vi "Min phase set (SubVI).vi"(3 "pos_z":dbl, 4 "error in":errorcluster, 5 "step search":i32=50, 6 "set_pos_min":dbl, 7 "VISA Refnum in":refnum<visa-resource-name>) -> (0 "error out":errorcluster, 1 "Min phase":dbl)   [LabVIEW 2018]
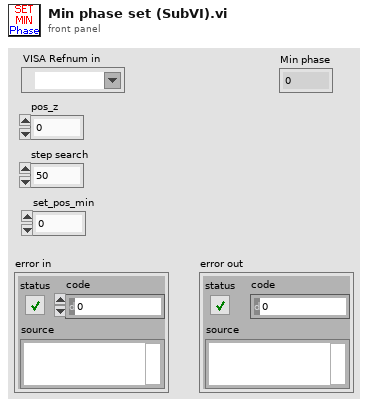
[diagram p1: front panel]
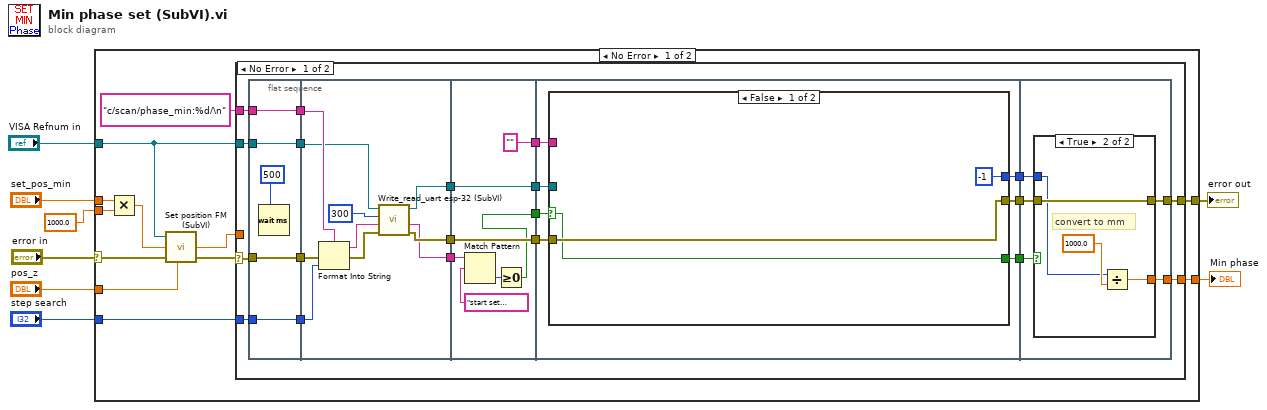
[diagram p0: block diagram]
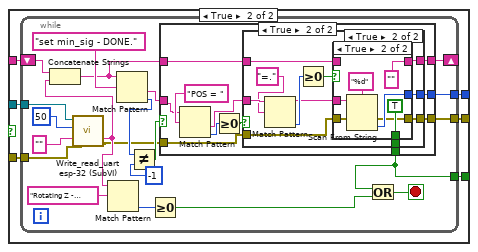
[diagram p2: hidden frame]
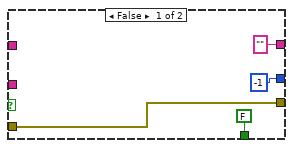
[diagram p3: hidden frame]
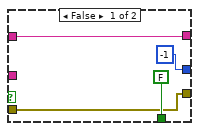
[diagram p4: hidden frame]
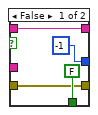
[diagram p5: hidden frame]
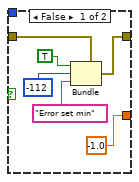
[diagram p6: hidden frame]
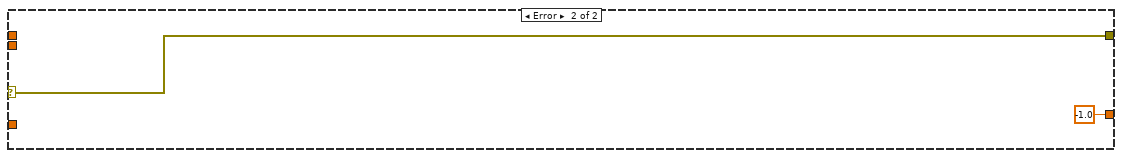
[diagram p8: hidden frame]
diagram:
  n1 = case shown="No Error" "error in" {
    selector: "error in" -> [w16 w159]
    tunnel: "VISA Refnum in" -> [w17 _]
    tunnel: [w20 w159] -> w8
    tunnel: [w19 -1.0] -> w5
    tunnel: "step search" -> [w18 _]
    tunnel: "pos_z" -> [w13 _]
    tunnel: "set_pos_min" -> [w12 _]
    tunnel: 1000.0 ("y") -> [w9 _]
    frame No Error {
      n2 = Multiply(x=w12, y=w9) -> (x*y=w11:dbl)
      n3 = call "Set position FM (SubVI).vi"("VISA Refnum in"=w17, "Позиция, мкм"=w11, "error in"=w16, "pos_z"=w13) -> ("set_pos_z"=w10:dbl, "error out"=w15:errorcluster)  [unwired: 2 in]
      n4 = case shown="No Error" w15 {
        selector: w15 -> [w25 w157]
        tunnel: "c/scan/phase_min:%d/\n" ("write buffer") -> [w30 _]
        tunnel: [w29 w157] -> w20
        tunnel: [w28 w156] -> w19
        tunnel: w18 -> [w27 _]
        tunnel: w17 -> [w26 _]
        tunnel: w10 -> [_ w156]
        frame No Error {
          n5 = flat-sequence {
            tunnel: w27 -> [w42]
            tunnel: w25 -> [w43]
            tunnel: w30 -> [w44]
            tunnel: w26 -> [w45]
            tunnel: [w45] -> w24
            tunnel: [w44] -> w23
            tunnel: [w43] -> w22
            tunnel: [w42] -> w21
            tunnel: [w54] -> w40
            tunnel: [w50] -> w39
            tunnel: [w47] -> w38
            tunnel: w24 -> [w48]
            tunnel: w23 -> [w49]
            tunnel: w22 -> [w51]
            tunnel: w21 -> [w46]
            tunnel: w40 -> [w62]
            tunnel: [w62] -> w37
            tunnel: w39 -> [w61]
            tunnel: [w61] -> w36
            tunnel: [w56] -> w35
            tunnel: w38 -> [w60]
            tunnel: ["" ("write buffer")] -> w34
            tunnel: w37 -> [w68]
            tunnel: w36 -> [w69]
            tunnel: w35 -> [w67]
            tunnel: [w66] -> w33
            tunnel: w34 -> [w65]
            tunnel: [w64] -> w32
            tunnel: [w63] -> w31
            tunnel: [w145] -> w29
            tunnel: w33 -> [w144]
            tunnel: w32 -> [w143]
            tunnel: w31 -> [w142]
            tunnel: [w141] -> w28
            frame #0 {
              n6 = Wait (ms)(milliseconds to wait=u32 500) -> ()  [unwired: 1 out]
            }
            frame #1 {
              n7 = Format Into String(format string=w49, error in=w51, w46) -> (resulting string=w53:string, error out=w52:errorcluster)  [unwired: 1 in]
              n8 = call "Write_read_uart esp-32 (SubVI).vi"("error in (no error)"=w52, "write buffer"=w53, "milliseconds to wait"=u32 300, "VISA Refnum in"=w48) -> ("error out 4"=w54:errorcluster, "read buffer"=w47:string, "VISA resource name out"=w50:refnum<visa-resource-name>)  [unwired: 1 out]
            }
            frame #2 {
              n9 = Match Pattern(string=w60, regular expression="start set minimum phase signal...") -> (offset past match=w58:i32)  [unwired: 1 in, 3 out]
              n10 = Greater Or Equal To 0?(x=w58) -> (x >= 0?=w56:bool)
            }
            frame #3 {
              n11 = case shown="False" w67 {
                selector: w67 -> [w70 _]
                tunnel: w68 -> [w71 w78]
                tunnel: w69 -> [_ w77]
                tunnel: [w70 w76] -> w66
                tunnel: w65 -> [_ w75]
                tunnel: [-1 w74] -> w64
                tunnel: [w71 w73] -> w63
                frame False {
                }
                frame True {
                  n12 = while {
                    tunnel: w78 -> [w97]
                    tunnel: w77 -> [w96]
                    tunnel: [w81] -> w76
                    shift-right: [w86] -> _
                    shift-left: w75 -> [w85]
                    tunnel: [w82] -> w74
                    tunnel: [w79] -> w73
                    stop <- w93 stop-if-true
                    n13 = call "Write_read_uart esp-32 (SubVI).vi"("error in (no error)"=w97, "write buffer"="", "milliseconds to wait"=u32 50, "VISA Refnum in"=w96) -> ("error out 4"=w80:errorcluster, "read buffer"=w84:string)  [unwired: 2 out]
                    n14 = Concatenate Strings(w85, w84) -> (w83:string)
                    n15 = Match Pattern(string=w84, regular expression="Rotating Z - stopped!") -> (offset past match=w90:i32)  [unwired: 1 in, 3 out]
                    n16 = Match Pattern(string=w83, regular expression="set min_sig - DONE.") -> (after substring=w87:string, offset past match=w92:i32)  [unwired: 1 in, 2 out]
                    n17 = Not Equal?(x=w92, y=-1 ("offset past match")) -> (x != y?=w88:bool)
                    n18 = Greater Or Equal To 0?(x=w90) -> (x >= 0?=w89:bool)
                    n19 = case shown="True" w88 {
                      tunnel: w87 -> [_ w110]
                      tunnel: w83 -> [_ w109]
                      tunnel: ["" ("read buffer") w108] -> w86
                      tunnel: [-1 w107] -> w82
                      tunnel: [FALSE w106] -> w81
                      tunnel: w80 -> [w100 w105]
                      tunnel: [w100 w104] -> w79
                      frame False {
                      }
                      frame True {
                        n20 = Match Pattern(string=w110, regular expression="POS = " ("write buffer")) -> (after substring=w111:string, offset past match=w113:i32)  [unwired: 1 in, 2 out]
                        n21 = Greater Or Equal To 0?(x=w113) -> (x >= 0?=w112:bool)
                        n22 = case shown="True" w112 {
                          tunnel: w111 -> [_ w129]
                          tunnel: w109 -> [w118 w124]
                          tunnel: [w118 w123] -> w108
                          tunnel: [-1 w122] -> w107
                          tunnel: [FALSE w121] -> w106
                          tunnel: w105 -> [w115 w120]
                          tunnel: [w115 w119] -> w104
                          frame False {
                          }
                          frame True {
                            n23 = Match Pattern(string=w129, regular expression="=." ("write buffer")) -> (before substring=w125:string, offset past match=w127:i32)  [unwired: 1 in, 2 out]
                            n24 = Greater Or Equal To 0?(x=w127) -> (x >= 0?=w126:bool)
                            n25 = case shown="True" w126 {
                              tunnel: w125 -> [_ w139]
                              tunnel: w124 -> [w133 _]
                              tunnel: [w133 "" ("read buffer")] -> w123
                              tunnel: [-1 w137] -> w122
                              tunnel: [FALSE TRUE] -> w121
                              tunnel: w120 -> [w130 w135]
                              tunnel: [w130 w134] -> w119
                              frame False {
                              }
                              frame True {
                                n26 = Scan From String(format string="%d", input string=w139, error in=w135) -> (error out=w134:errorcluster, output 1=w137:i32)  [unwired: 2 in, 2 out]
                              }
                            }
                          }
                        }
                      }
                    }
                    n27 = Or(x=w81, y=w89) -> (x .or. y?=w93:bool)
                  }
                }
              }
            }
            frame #4 {
              n28 = case shown="True" w144 {
                tunnel: w142 -> [w150 w155]
                tunnel: [w147 w155] -> w145
                tunnel: w143 -> [_ w153]
                tunnel: [-1.0 w152] -> w141
                frame False {
                  n29 = Bundle(cluster=w150, "status"=TRUE, "code"=-112, "source"="Error set min") -> (w147:errorcluster)
                }
                frame True {
                  # "convert to mm"
                  n30 = Divide(x=w153, y=1000.0 ("x")) -> (x/y=w152:dbl)
                }
              }
            }
          }
        }
        frame Error {
        }
      }
    }
    frame Error {
    }
  }
  "error out" <- w8
  "Min phase" <- w5
